vi "Monitor Ready For Start Condition.vi"(0 "channel status":T1, 5 "configuration":T3) -> (4 "ready for start":bool)   [LabVIEW 2020, in "GettingStarted_Gen_148X_FPGA.lvlib"]
uses:
  GettingStarted_Gen_148X_FPGA.lvlib
  Types/Serial Output Channel Datapath Configuration.ctl
  Types/Serial Output Channel Status.ctl
  Common/Types/DRAM Status.ctl
  Common/GettingStarted_Common_148X_FPGA.lvlib
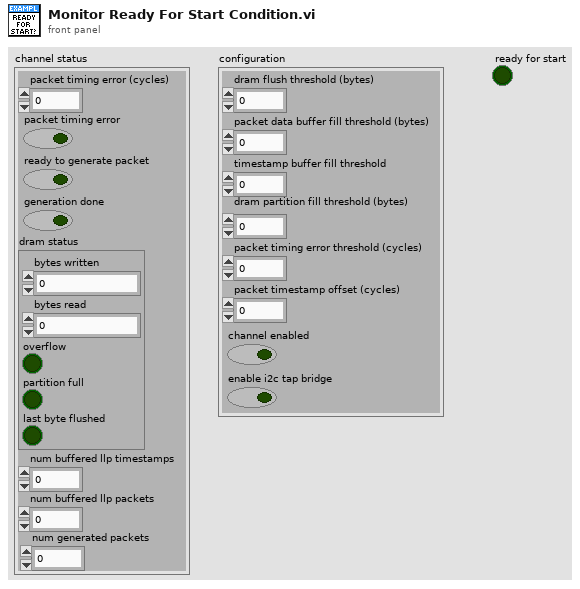
[diagram p1: front panel]
types:
  T1 = typedef "GettingStarted_Gen_148X_FPGA.lvlib/Serial Output Channel Status.ctl" = cluster{"num buffered llp packets":fxp<+,14,14>, "packet timing error (cycles)":u64, "packet timing error":bool, "ready to generate packet":bool, "dram status":T2, "num buffered llp timestamps":u32, "generation done":bool, "num generated packets":u64}
  T2 = typedef "GettingStarted_Common_148X_FPGA.lvlib/DRAM Status.ctl" = cluster{"bytes written":u64, "bytes read":u64, "overflow":bool, "partition full":bool, "last byte flushed":bool}
  T3 = typedef "GettingStarted_Gen_148X_FPGA.lvlib/Serial Output Channel Datapath Configuration.ctl" = cluster{"dram flush threshold (bytes)":u64, "packet data buffer fill threshold (bytes)":u64, "timestamp buffer fill threshold":u32, "packet timing error threshold (cycles)":u64, "channel enabled":bool, "dram partition fill threshold (bytes)":u64, "enable i2c tap bridge":bool, "packet timestamp offset (cycles)":i64}
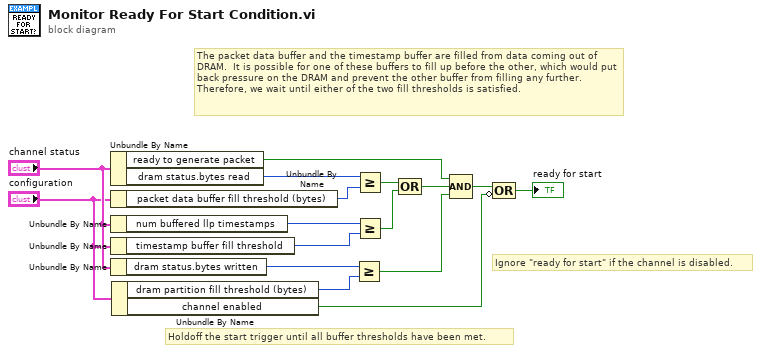
[diagram p0: block diagram]
diagram:
  # "The packet data buffer and the timestamp buffer are filled from data coming out of DRAM.  It is possible for one of these buffers to fill up before the other, which would put back pressure on the DRAM and prevent the other buffer from filling any further.  Therefore, we wait until either of the two fill thresholds is satisfied."
  # "Holdoff the start trigger until all buffer thresholds have been met."
  # "Ignore \"ready for start\" if the channel is disabled."
  n1 = Unbundle By Name("channel status") -> ("ready to generate packet"=w12:bool, "dram status.bytes read"=w10:u64)
  n2 = Unbundle By Name("configuration") -> ("packet data buffer fill threshold (bytes)"=w13:u64)
  n3 = Unbundle By Name("channel status") -> ("num buffered llp timestamps"=w11:u32)
  n4 = Unbundle By Name("configuration") -> ("timestamp buffer fill threshold"=w14:u32)
  n5 = Unbundle By Name("channel status") -> ("dram status.bytes written"=w4:u64)
  n6 = Unbundle By Name("configuration") -> ("dram partition fill threshold (bytes)"=w7:u64, "channel enabled"=w5:bool)
  n7 = Greater Or Equal?(x=w4, y=w7) -> (x >= y?=w6:bool)
  n8 = Greater Or Equal?(x=w10, y=w13) -> (x >= y?=w2:bool)
  n9 = Greater Or Equal?(x=w11, y=w14) -> (x >= y?=w3:bool)
  n10 = Compound Arithmetic op=OR(w2, w3) -> (w1:bool)
  n11 = Compound Arithmetic op=AND(w12, w1, w6) -> (w15:bool)
  n12 = Compound Arithmetic op=OR(w15, invert w5) -> (→"ready for start":bool)
